vi "Read Configuration Version.vi"(8 "error in (no error)":errorcluster, 11 "dsf refnum":T2) -> (0 "error out":errorcluster, 2 "version":T1, 3 "dsf refnum out":T2)   [LabVIEW 2017, in "DSF Core.lvlib"]
doc: "Reads a value associated with a key in a specified section from the configuration data identified by <B>dsf refnum</B>. If the key does not exist, the VI returns the default value. This VI supports multibyte characters in strings. Wire data to the <B>default value</B> input to determine the polymorphic instance to use or manually select the instance."
uses:
  DSF Core.lvlib
  Public/Controls/DSF Config Data RefNum.ctl
  Public/Controls/DSF Version Info.ctl
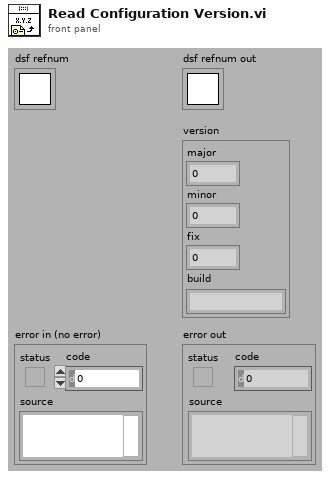
[diagram p1: front panel]
types:
  T1 = typedef "DSF Core.lvlib/DSF Version Info.ctl" = cluster{"major":u32, "minor":u32, "fix":u32, "build":string}
  T2 = typedef "DSF Core.lvlib/DSF Config Data RefNum.ctl" = refnum<k1>
  T3 = typedef "DSF Core.lvlib/DSF Configuration Reference.ctl" = refnum<data-value>
  T4 = typedef "DSF Core.lvlib/Internal.DSF Configuration.ctl" = cluster{"dsfversion":T1, "version":T1, "plugins":T5[], "groups":T8[], "transfers":T10[], "channels":T12[], "settings":T14[]}
  T5 = typedef "DSF Core.lvlib/Internal.DSF Plugin with ID.ctl" = cluster{"id":string, "values":T6}
  T6 = typedef "DSF Core.lvlib/Internal.DSF Plugin Info.ctl" = cluster{"type":string, "timing":T7, "group ids":string[], "settings id":string}
  T7 = typedef "DSF Core.lvlib/DSF Timing Info.ctl" = cluster{"priority":u64, "decimation":u64, "offset":u64}
  T8 = typedef "DSF Core.lvlib/Internal.DSF Group with ID.ctl" = cluster{"id":string, "values":T9}
  T9 = typedef "DSF Core.lvlib/Internal.DSF Group Info.ctl" = cluster{"direction":i32, "timing":T7, "transfer ids":string[], "settings id":string}
  T10 = typedef "DSF Core.lvlib/Internal.DSF Transfer with ID.ctl" = cluster{"id":string, "values":T11}
  T11 = typedef "DSF Core.lvlib/Internal.DSF Transfer Info.ctl" = cluster{"byte order":i32, "channel ids":string[], "settings id":string}
  T12 = typedef "DSF Core.lvlib/Internal.DSF Channel with ID.ctl" = cluster{"id":string, "values":T13}
  T13 = typedef "DSF Core.lvlib/Internal.DSF Channel Info.ctl" = cluster{"count":u64, "buffer offset":u64, "data type":i32, "settings id":string}
  T14 = typedef "DSF Core.lvlib/Internal.DSF Settings with ID.ctl" = cluster{"id":string, "values":T15}
  T15 = typedef "DSF Core.lvlib/Internal.DSF Settings Info.ctl" = cluster{"key":string, "value":string}[]
  T16 = cluster{"dsf configuration":T4, "path":path, "dirty":bool}
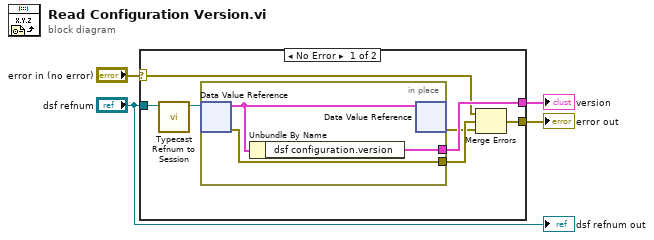
[diagram p0: block diagram]
diagram:
  n1 = case shown="No Error" "error in (no error)" {
    selector: "error in (no error)" -> [w7 w15]
    tunnel: "dsf refnum" -> [w11 _]
    tunnel: [w8 w15] -> w2
    tunnel: [w9 _] -> w3
    frame No Error {
      n2 = call "Typecast Refnum to Session.vi"("dsf refnum in"=w11) -> ("DSF Configuration Session out"=w10:T3)  [unwired: 10 in]
      n3 = in-place {
        in-place-border: [w14] -> w9
        in-place-border: [w13] -> w6
        n4 = in-place-dvr #1(w10) -> (w12:T16, w13:errorcluster)
        n5 = Unbundle By Name(w12) -> ("dsf configuration.version"=w14:T1)
        n6 = in-place-dvr #1(w12) -> (w5:errorcluster)  [unwired: 1 out]
      }
      n7 = Merge Errors(w7, w6, w5) -> (w8:errorcluster)
    }
    frame Error {
    }
  }
  "error out" <- w2
  "version" <- w3
  "dsf refnum out" <- "dsf refnum"
